vi "ProtocolAnalysis.vi"(8 "error in":errorcluster caption="错误输入", 11 "TCP ref in":refnum<k5>) -> (0 "error out":errorcluster caption="错误输出", 2 "Exit":bool, 3 "TCP ref out":refnum<k5>, 4 "55":string, 5 "AA":string)   [LabVIEW 2014]
panel:
  out "string":string
  out "01":u8
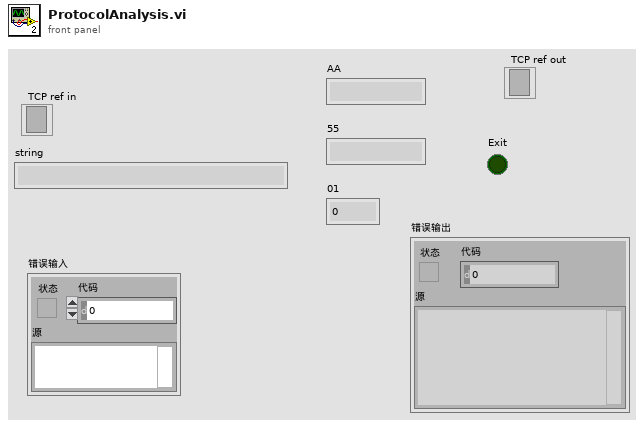
[diagram p1: front panel]
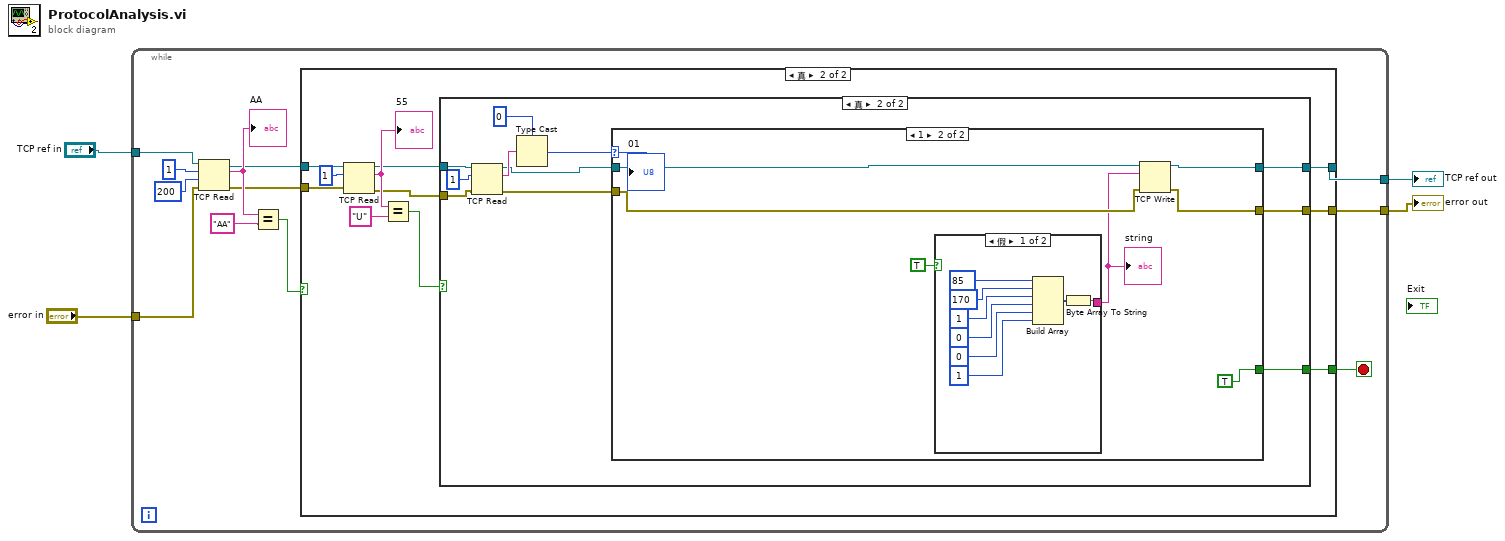
[diagram p0: block diagram]
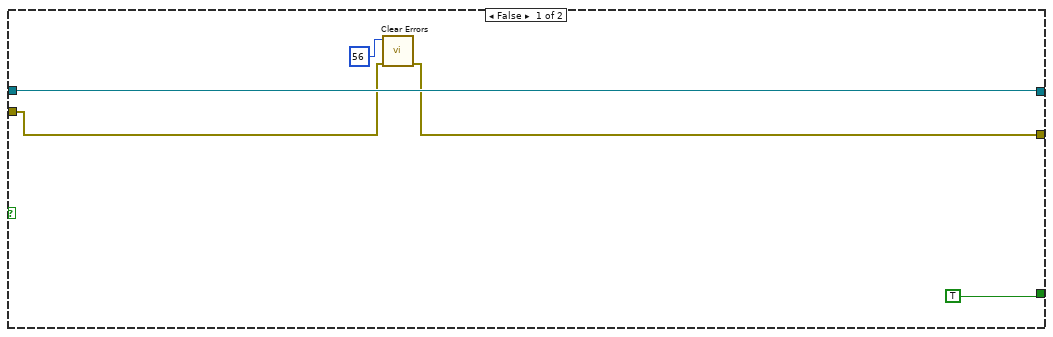
[diagram p2: hidden frame]
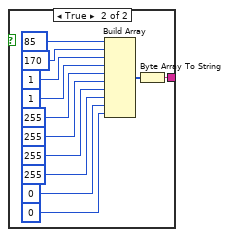
[diagram p5: hidden frame]
diagram:
  n1 = while {
    tunnel: "TCP ref in" -> [w16]
    tunnel: "error in" -> [w15]
    tunnel: [w7] -> w2
    tunnel: [w6] -> w1
    stop <- w5 stop-if-true
    n2 = TCP Read(connection ID=w16, bytes to read=1 ("读取的字节"), error in (no error)=w15, 9:200 ("超时毫秒(25000)")) -> (connection ID out=w9:refnum<k5>, data out=w12:string, error out=w8:errorcluster)  [unwired: 1 in]
    "AA" <- w12
    n3 = Equal?(x=w12, y="AA") -> (x = y?=w10:bool)
    n4 = case shown="真" w10 {
      tunnel: w9 -> [w21 w29]
      tunnel: w8 -> [w19 w28]
      tunnel: [w21 w24] -> w7
      tunnel: [w18 w23] -> w6
      tunnel: [TRUE w22] -> w5
      frame False {
        n5 = call <vilib>:"Clear Errors.vi"("error in (no error)"=w19, "specific error code to clear (0: all)"=56) -> ("error out"=w18:errorcluster)  [unwired: 4 in, 1 out]
      }
      frame True {
        n6 = TCP Read(connection ID=w29, bytes to read=1 ("读取的字节"), error in (no error)=w28) -> (connection ID out=w25:refnum<k5>, data out=w31:string, error out=w26:errorcluster)  [unwired: 2 in]
        "55" <- w31
        n7 = Equal?(x=w31, y="U") -> (x = y?=w27:bool)
        n8 = case shown="真" w27 {
          tunnel: w26 -> [w33 w42]
          tunnel: w25 -> [w34 w41]
          tunnel: [w34 w38] -> w24
          tunnel: [w33 w37] -> w23
          tunnel: [_ w35] -> w22
          frame False {
          }
          frame True {
            n9 = TCP Read(connection ID=w41, bytes to read=1 ("读取的字节"), error in (no error)=w42) -> (connection ID out=w39:refnum<k5>, data out=w44:string, error out=w36:errorcluster)  [unwired: 2 in]
            n10 = Type Cast(type=u8 0, x=w44) -> (*(type *) &x=w40:u8)
            n11 = case shown="1" w40 {
              selector: w40 -> [_ w48]
              tunnel: w39 -> [w47 w55]
              tunnel: [w47 w54] -> w38
              tunnel: [w46 w52] -> w37
              tunnel: w36 -> [w46 w53]
              tunnel: [_ TRUE] -> w35
              frame 0, Default {
              }
              frame 1 {
                n12 = case shown="假" TRUE {
                  tunnel: [w56 w64] -> w51
                  frame False {
                    n13 = Build Array(u8 85, u8 170, u8 1, u8 0, u8 0, u8 1) -> (w57:u8[])
                    n14 = Byte Array To String(unsigned byte array=w57) -> (string=w56:string)
                  }
                  frame True {
                    n15 = Build Array(u8 85, u8 170, u8 1, u8 1, u8 255, u8 255, u8 255, u8 255, u8 0, u8 0) -> (w65:u8[])
                    n16 = Byte Array To String(unsigned byte array=w65) -> (string=w64:string)
                  }
                }
                "string" <- w51
                n17 = TCP Write(connection ID=w55, data in=w51, error in (no error)=w53) -> (connection ID out=w54:refnum<k5>, error out=w52:errorcluster)  [unwired: 1 in, 1 out]
                "01" <- w48
              }
            }
          }
        }
      }
    }
  }
  "error out" <- w1
  "TCP ref out" <- w2
